vi "GetPressure.vi"(8 "error in (no error)":errorcluster, 11 "IGauge in":refnum<class "IGauge.lvclass">) -> (0 "error out":errorcluster, 2 "Pressure (mbar)":dbl, 3 "IGauge out":refnum<class "IGauge.lvclass">)   [LabVIEW 2016, in "IGauge.lvlib" / "IGauge.lvclass"]
uses:
  IGauge.lvclass
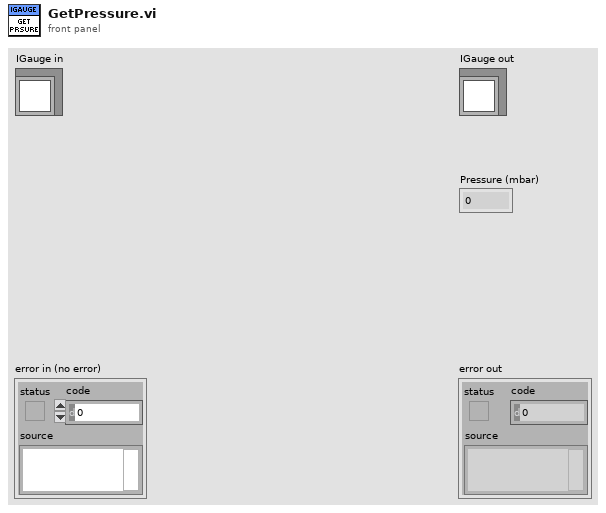
[diagram p1: front panel]
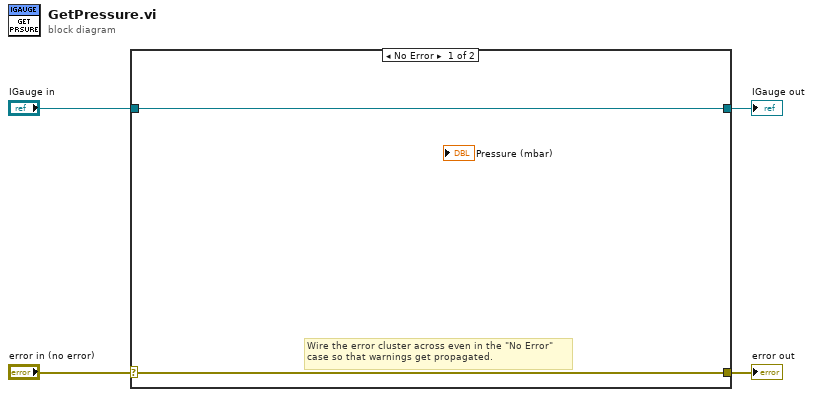
[diagram p0: block diagram]
diagram:
  n1 = case shown="No Error" "error in (no error)" {
    selector: "error in (no error)" -> [w5 w8]
    tunnel: [w5 w8] -> w3
    tunnel: [w6 w7] -> w1
    tunnel: "IGauge in" -> [w6 w7]
    frame No Error {
      # "Wire the error cluster across even in the \"No Error\"\ncase so that warnings get propagated."
    }
    frame Error {
    }
  }
  "error out" <- w3
  "IGauge out" <- w1
